vi "TCP-Cllient_.vi"() -> ()   [LabVIEW 2020]
doc: "演示连接TCP服务器、读取发送的数据并在图表上显示数据的方法。VI设计为TCP连接断开时停止。"
panel:
  out "波形图表 3":i32[](graph)
  in  "file path (dialog if empty)":path caption="文件路径 （空时为对话框）"
  in  "服务器关闭":string="服务器VI关闭了连接。"
  in  "停止":bool
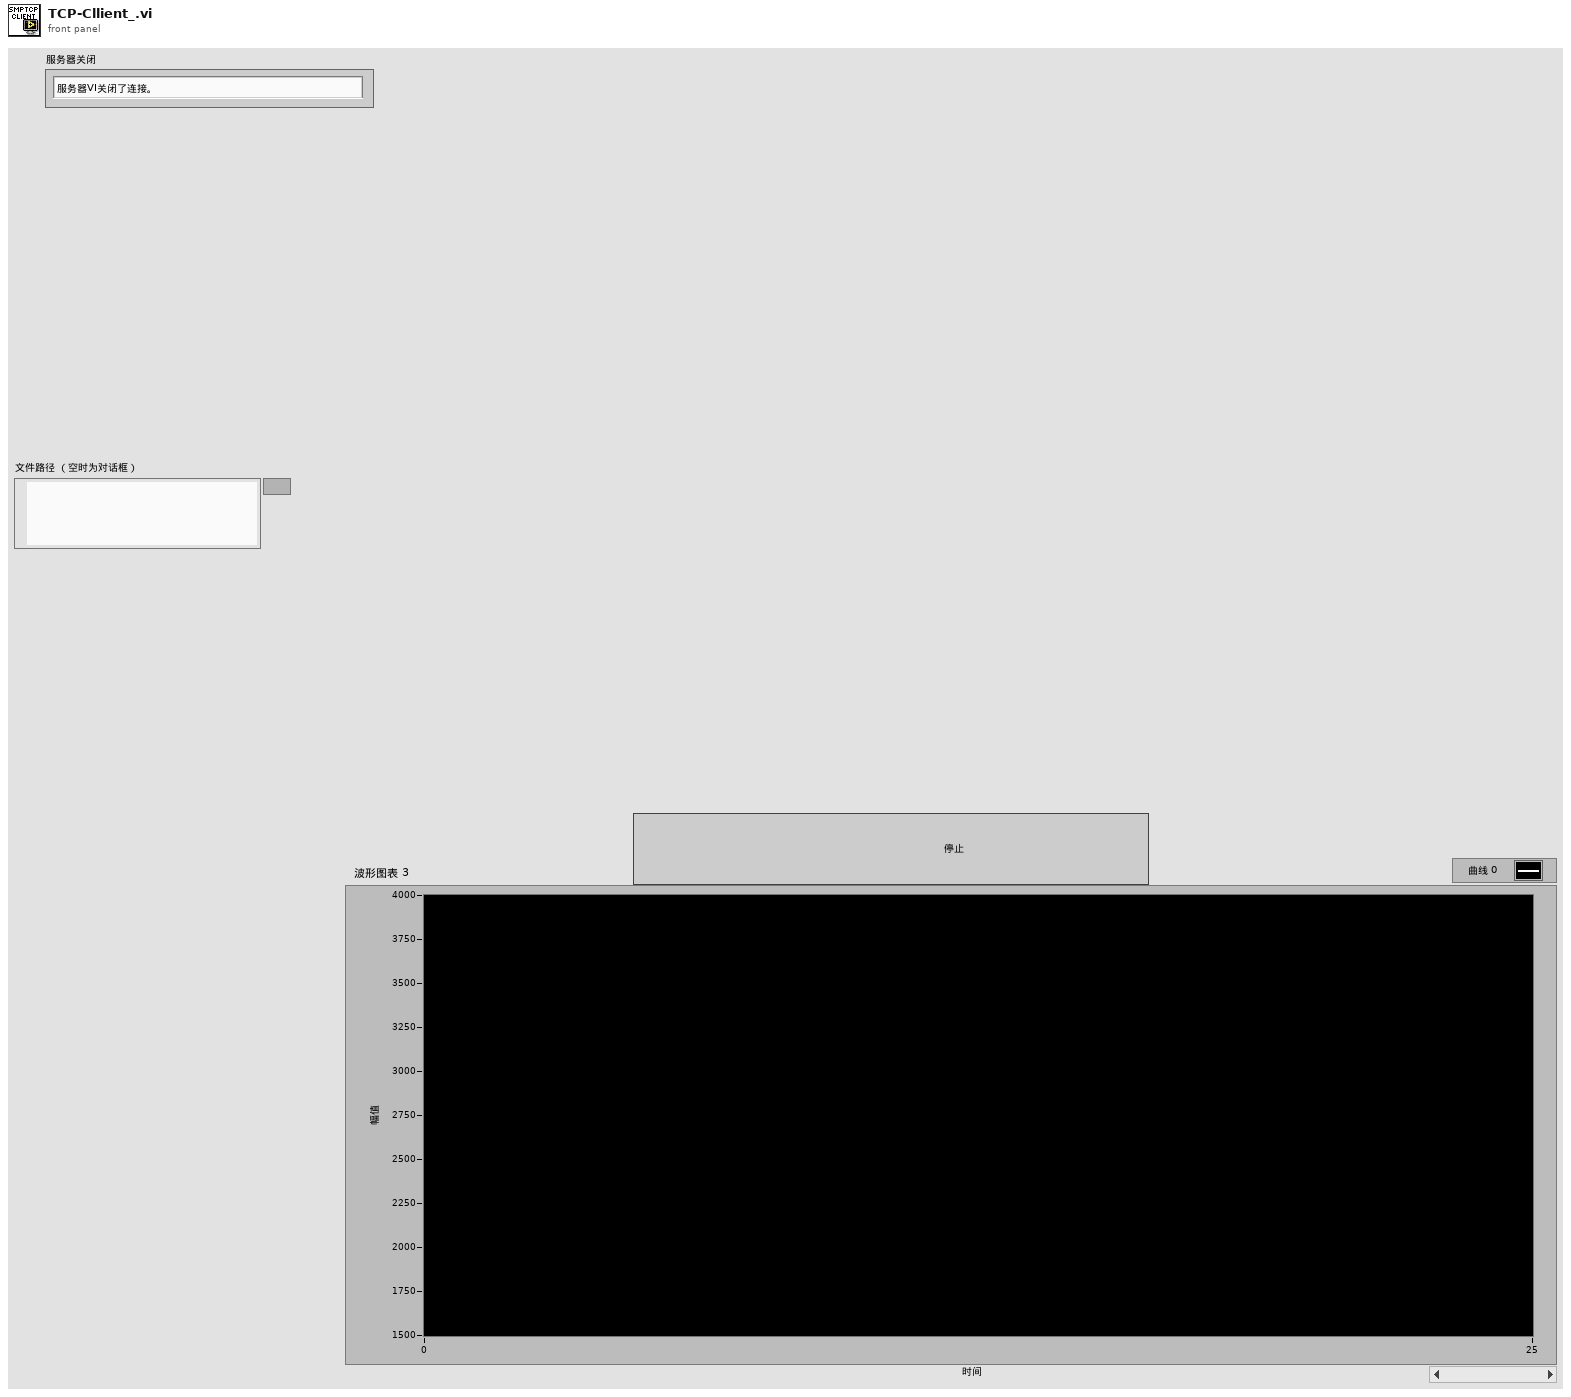
[diagram p1: front panel]
types:
  T1 = enum16{"open", "open or create", "create or replace", "create", "open (read-only)"}
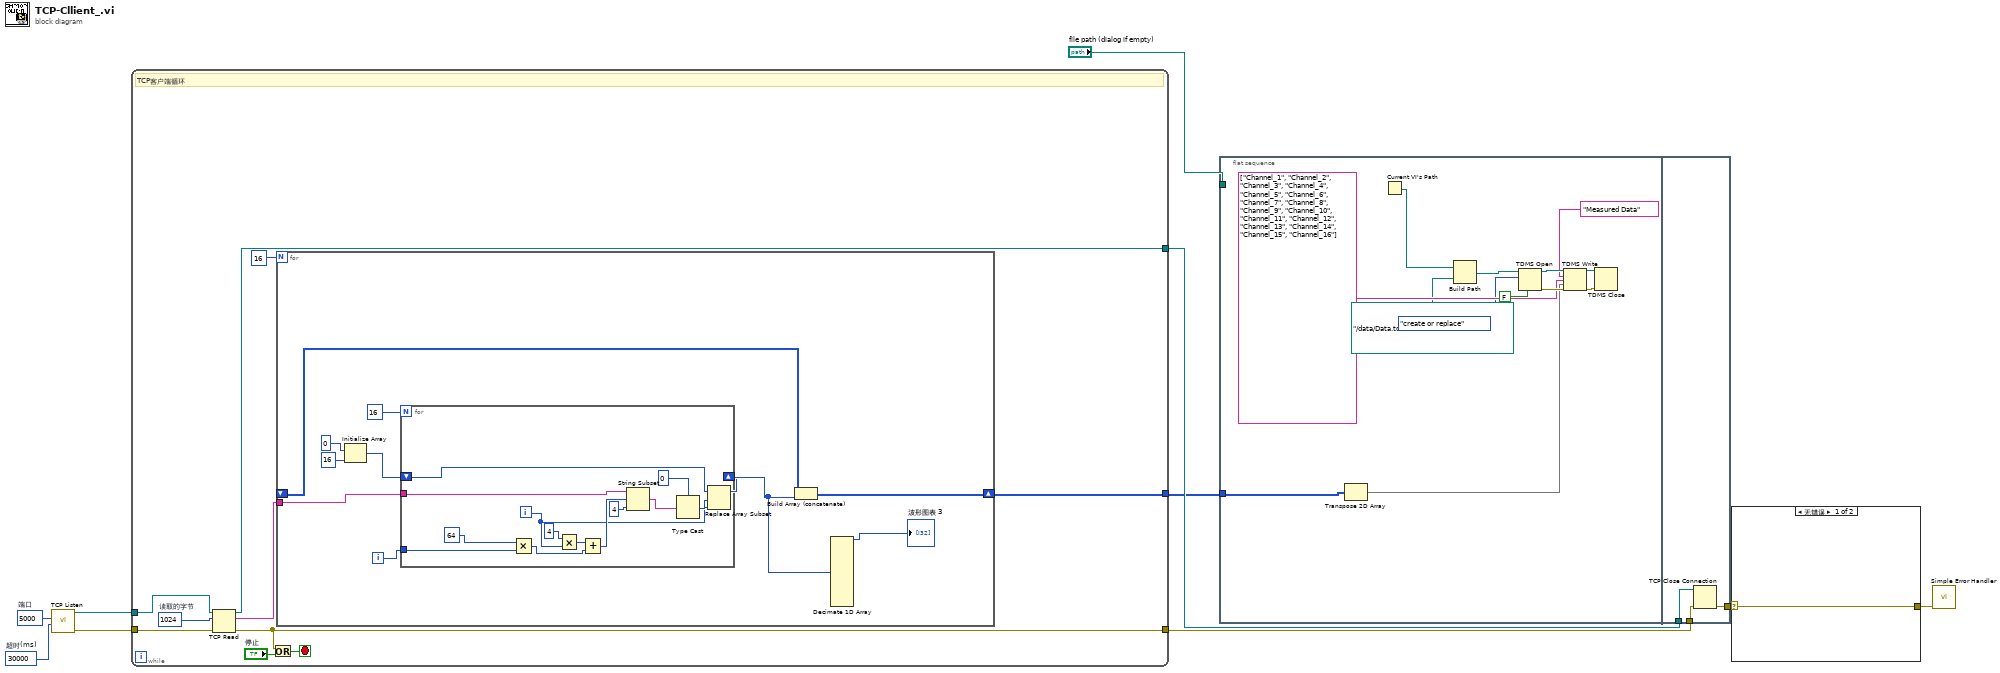
[diagram p0: block diagram]
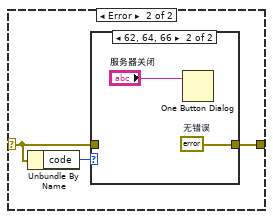
[diagram p2: hidden frame]
diagram:
  w6 = u16 5000  # 端口
  w9 = 30000  # 超时(ms)
  n1 = call <vilib>:"TCP Listen.vi"("timeout ms (wait forever: -1)"=w9, "port"=w6) -> ("error out"=w7:errorcluster, "connection ID"=w8:refnum<k5>)  [unwired: 5 in, 3 out]
  n2 = while {
    tunnel: w7 -> [w19]
    tunnel: w8 -> [w20]
    tunnel: [w16] -> w3
    tunnel: [w15] -> w4
    tunnel: [w11] -> w1
    stop <- w17 stop-if-true
    w14 = 1024  # 读取的字节
    # "TCP客户端循环"
    n3 = TCP Read(connection ID=w20, bytes to read=w14, error in (no error)=w19) -> (connection ID out=w16:refnum<k5>, data out=w13:string, error out=w15:errorcluster)  [unwired: 2 in]
    n4 = Or(x=w15, y="停止") -> (x .or. y?=w17:bool)
    n5 = for {
      N: u8 16 -> [_]
      tunnel: w13 -> [w30]
      shift-right: [w24] -> w11
      shift-left: _ -> [w23]
      i -> [w25]
      n6 = Initialize Array(0, 16) -> (w26:i32[])
      n7 = for {
        N: i8 16 -> [_]
        tunnel: w30 -> [w42]
        tunnel: w25 -> [w38]
        shift-right: [w31] -> w21
        shift-left: w26 -> [w32]
        i -> [w33]
        n8 = Multiply(x=i8 64, y=w38) -> (x*y=w37:i32)
        n9 = Multiply(x=i8 4, y=w33) -> (x*y=w35:i32)
        n10 = Add(x=w35, y=w37) -> (x+y=w36:i32)
        n11 = String Subset(string=w42, offset (0)=w36, length (rest)=i8 4) -> (substring=w44:string)
        n12 = Type Cast(type=0, x=w44) -> (*(type *) &x=w34:i32)
        n13 = Replace Array Subset(array=w32, new element=w34, index=w33) -> (w31:i32[])
      }
      n14 = Build Array (concatenate)(w23, w21) -> (w24:i32[][])
      n15 = Decimate 1D Array(w21) -> (→"波形图表 3":i32[])  [unwired: 11 out]
    }
  }
  n16 = flat-sequence {
    tunnel: "file path (dialog if empty)" -> [_]
    tunnel: w1 -> [w47]
    tunnel: w4 -> [w60]
    tunnel: w3 -> [w59]
    tunnel: [w58] -> w2
    frame #0 {
      n17 = Transpose 2D Array(2D array=w47) -> (transposed array=w46:i32[][])
      n18 = Current VI's Path() -> (path=w45:path)
      n19 = Build Path(base path=w45, name or relative path=path "../data/Data.tdms" ("file path")) -> (appended path=w53:path)
      n20 = TDMS Open(6:FALSE ("disable buffering (T)"), 10:T1."create or replace" ("operation"), 11:w53) -> (0:w57:errorcluster, 3:w54:refnum<k34>)  [unwired: 4 in]
      n21 = TDMS Write(0:w54, 5:"Measured Data" ("group name"), 7:string[] ["Channel_1", "Channel_2", "Channel_3", "Channel_4", "Channel_5", "Channel_6", "Channel_7", "Channel_8", "Channel_9", "Channel_10", "Channel_11", "Channel_12", "Channel_13", "Channel_14", "Channel_15", "Channel_16"] ("channel names"), 9:w46, 11:w57) -> (4:w55:refnum<k34>, 15:w56:errorcluster)  [unwired: 1 in, 2 out]
      n22 = TDMS Close(8:w56, 11:w55) -> ()  [unwired: 2 out]
    }
    frame #1 {
      n23 = TCP Close Connection(connection ID=w59, error in (no error)=w60) -> (error out=w58:errorcluster)  [unwired: 1 in, 1 out]
    }
  }
  n24 = case shown="无错误" w2 {
    selector: w2 -> [w61 w63]
    tunnel: [w61 w62] -> w10
    frame No Error {
    }
    frame Error {
      n25 = Unbundle By Name(w63) -> ("code"=w64:i32)
      n26 = case shown="62, 64, 66" w64 {
        tunnel: w63 -> [w65 _]
        tunnel: [w65 w67] -> w62
        frame Default {
        }
        frame 62, 64, 66 {
          w67 = errorcluster {"status"=FALSE, "code"=0, "source"=""}  # 无错误
          n27 = One Button Dialog(message="服务器关闭") -> ()  [unwired: 1 in, 1 out]
        }
      }
    }
  }
  n28 = call <vilib>:"Simple Error Handler.vi"("error in (no error)"=w10) -> ()  [unwired: 4 in, 5 out]
